vi "UpdateClassVIsConnectorPattern.vi"(0 "ClassRefIn":refnum<vi>, 5 "error in (no error)":errorcluster, 6 "ClassWriter in":refnum<class "ClassWriter.lvclass">) -> (12 "ClassWriter out":refnum<class "ClassWriter.lvclass">, 14 "ClassRefOut":refnum<vi>, 19 "error out":errorcluster)   [LabVIEW 2012, in "ClassWriter.lvclass"]
uses:
  <resource>/Framework/Providers/Open_GDS/ClassProviders/Provider_BaseClassInterface/ClassWriter_class/ClassWriter.lvclass
  <resource>/Framework/Providers/Open_GDS/ClassProviders/Common/ScriptingFunctions/Scripting_ConnectorPanePatternType.ctl
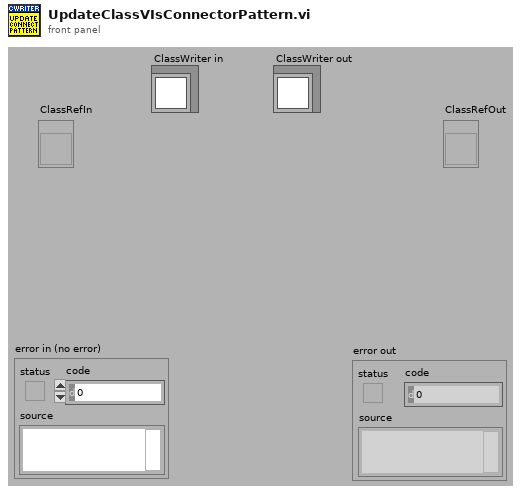
[diagram p1: front panel]
types:
  T1 = typedef "Scripting_ConnectorPanePatternType.ctl" = u16
  T2 = typedef "GDSLvCLass_ClassSettingsType.ctl" = cluster{"ClassProviderName":string, "ClassTemplateUsed":string, "ClassTemplateVersion":string, "ClassDescription":string, "PlugIns":T3[], "ConnectorPanePattern":string}
  T3 = typedef "GDSLvClass_PlugIn.ctl" = cluster{"Type":T4, "ID":string, "Version":string, "Path":path, "Name":string, "Data":variant}
  T4 = typedef "GDSLvClass_PlugInTypes.ctl" = enum16{"DesignPattern", "MethodTypes"}
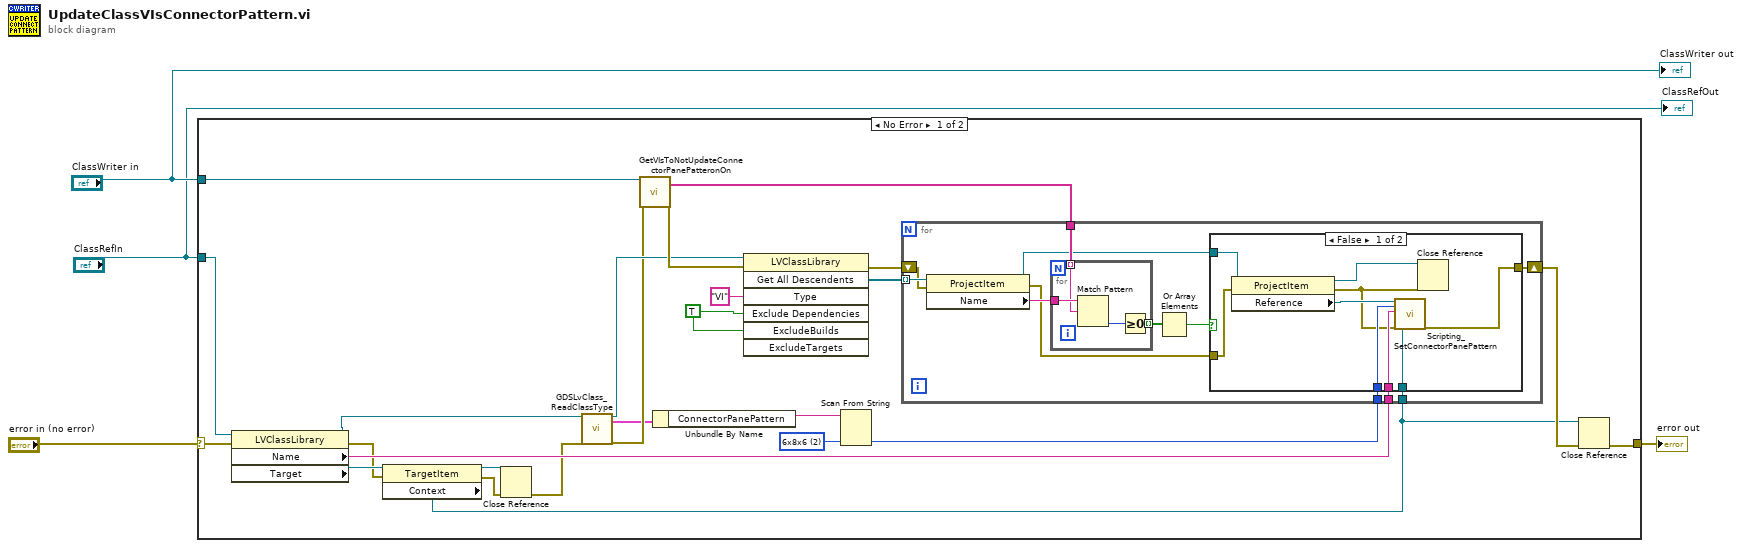
[diagram p0: block diagram]
diagram:
  n1 = case shown="No Error" "error in (no error)" {
    selector: "error in (no error)" -> [w13 w56]
    tunnel: "ClassRefIn" -> [w17 _]
    tunnel: "ClassWriter in" -> [w26 _]
    tunnel: [w5 w56] -> w1
    frame No Error {
      w19 = T1 2 items=["4x4x4", "5x6x5", "6x8x6"] ("Pattern")
      w14 = TRUE ("ExcludeDependencies")
      n2 = property class="LVClassLibrary"(reference=w17, error in=w13) -> (reference out=w16:refnum<vi>, error out=w10:errorcluster, "Name"=w15:string, "Target"=w12:refnum<vi>)
      n3 = property class="TargetItem"(reference=w12, error in=w10) -> (reference out=w11:refnum<vi>, error out=w8:errorcluster, "Context"=w6:refnum<vi>)
      n4 = Close Reference(reference=w11, error in (no error)=w8) -> (error out=w9:errorcluster)
      n5 = call <resource>:"GDSLvClass_ReadClassType.vi"("Class Refnum In"=w16, "error in (no error)"=w9) -> ("Class Refnum Out"=w23:refnum<vi>, "ClassSettings"=w21:T2, "error out"=w22:errorcluster)  [unwired: 15 in]
      n6 = call-dynamic "GetVIsToNotUpdateConnectorPanePatteronOn.vi"("ClassWriter in"=w26, "error in (no error)"=w22) -> ("VIsToNotUpdateConnectorPanePatteronOn"=w25:string[], "error out"=w27:errorcluster)  [unwired: 15 in, 1 out]
      n7 = Unbundle By Name(w21) -> ("ConnectorPanePattern"=w20:string)
      n8 = invoke class="LVClassLibrary" method="Get All Descendents"(reference=w23, error in=w27, "Type"="VI", "Exclude Dependencies"=w14, "ExcludeBuilds"=w14) -> (error out=w24:errorcluster, "All Descendents"=w28:refnum<vi>[])  [unwired: 2 in, 5 out]
      n9 = Scan From String(input string=w20, default 1=w19) -> (output 1=w18:T1)  [unwired: 3 in, 3 out]
      n10 = for {
        tunnel: w28 -> [w41] mode=indexing
        tunnel: w25 -> [w39]
        shift-right: [w33] -> w7
        shift-left: w24 -> [w34]
        tunnel: w18 -> [w32]
        tunnel: w15 -> [w31]
        tunnel: w6 -> [w30]
        n11 = property class="ProjectItem"(reference=w41, error in=w34) -> (reference out=w36:refnum<vi>, error out=w35:errorcluster, "Name"=w40:string)
        n12 = for {
          tunnel: w40 -> [w55]
          tunnel: w39 -> [w54] mode=indexing
          tunnel: [w52] -> w38 mode=indexing
          n13 = Match Pattern(string=w55, regular expression=w54) -> (offset past match=w53:i32)  [unwired: 1 in, 3 out]
          n14 = Greater Or Equal To 0?(x=w53) -> (x >= 0?=w52:bool)
        }
        n15 = Or Array Elements(Boolean array=w38) -> (logical OR=w37:bool)
        n16 = case shown="False" w37 {
          tunnel: w36 -> [w50 _]
          tunnel: w35 -> [w48 w51]
          tunnel: [w47 w51] -> w33
          tunnel: w32 -> [w46 _]
          tunnel: w31 -> [w45 _]
          tunnel: w30 -> [w42 _]
          frame False {
            n17 = property class="ProjectItem"(reference=w50, error in=w48) -> (reference out=w43:refnum<vi>, error out=w44:errorcluster, "Reference"=w49:refnum<vi>)
            n18 = call <resource>:"Scripting_SetConnectorPanePattern.vi"("VIPath(s)/ViRef(s)"=w49, "Pattern"=w46, "UpdateCallersInThisClassOnly"=w45, "error in (no error)"=w44, "AppRef"=w42) -> ("error out"=w47:errorcluster)  [unwired: 14 in]
            n19 = Close Reference(reference=w43, error in (no error)=w44) -> ()  [unwired: 1 out]
          }
          frame True {
          }
        }
      }
      n20 = Close Reference(reference=w6, error in (no error)=w7) -> (error out=w5:errorcluster)
    }
    frame Error {
    }
  }
  "error out" <- w1
  "ClassRefOut" <- "ClassRefIn"
  "ClassWriter out" <- "ClassWriter in"
